vi "Execute.vi"(6 "Error":errorcluster, 7 "Message":refnum<class "Message.lvclass">, 11 "Actor":refnum<class "Actor.lvclass">) -> (3 "Actor":refnum<class "Actor.lvclass">, 4 "Error":errorcluster, 5 "Message":refnum<class "Message.lvclass">)   [LabVIEW 2020, in "jettl.lvlib" / "Message.lvclass"]
uses:
  Message.lvclass
  Actor/Actor.lvclass
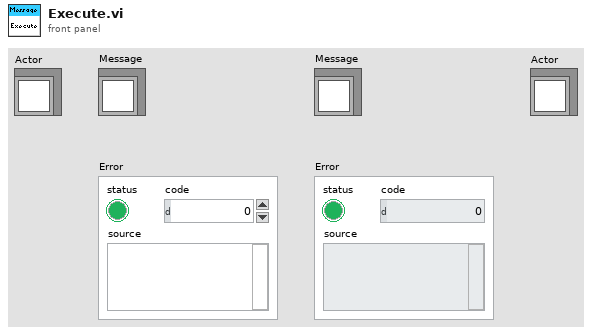
[diagram p1: front panel]
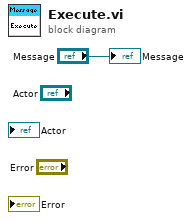
[diagram p0: block diagram]
diagram:
  "Message" <- "Message"
